vi "BPM.vi"(6 "threshold":i32, 8 "bpm":i32, 9 "fallingEdge":bool=TRUE, 10 "risingEdge":bool=TRUE, 11 "signal":i32) -> (0 "outBPM":i32, 1 "risingEdge_out":bool, 2 "fallingEdge_out":bool, 3 "outSignal":i32)   [LabVIEW 2014]
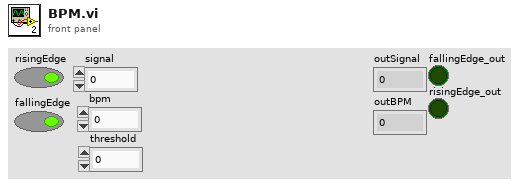
[diagram p1: front panel]
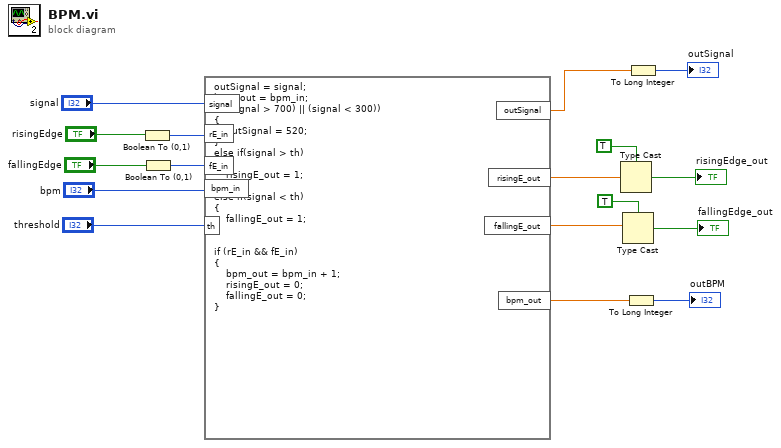
[diagram p0: block diagram]
diagram:
  n1 = Boolean To (0,1)(Boolean="risingEdge") -> (0, 1=w14:i16)
  n2 = Boolean To (0,1)(Boolean="fallingEdge") -> (0, 1=w16:i16)
  n3 = formula code="outSignal = signal;\nbpm_out = bpm_in;\nif ((signal > 700) || (signal < 300))\n{\n    outSignal = 520;\n}\nelse if(signal > th)\n{\n    risingE_out = 1;\n}\nelse if(signal < th)\n{\n    fallingE_out = 1;\n}\n\nif (rE_in && fE_in)\n{\n    bpm_out = bpm_in + 1;\n    risingE_out = 0;\n    fallingE_out = 0;\n}"("signal"="signal", "rE_in"=w14, "fE_in"=w16, "bpm_in"="bpm", "th"="threshold") -> ("outSignal"=w11:dbl, "risingE_out"=w7:dbl, "fallingE_out"=w6:dbl, "bpm_out"=w9:dbl)
  n4 = Type Cast(type=TRUE, x=w7) -> (*(type *) &x=→"risingEdge_out":bool)
  n5 = Type Cast(type=TRUE, x=w6) -> (*(type *) &x=→"fallingEdge_out":bool)
  n6 = To Long Integer(number=w9) -> (32bit integer=→"outBPM":i32)
  n7 = To Long Integer(number=w11) -> (32bit integer=→"outSignal":i32)
